vi "Redraw full indicator.vi"(8 "error in (no error)":errorcluster, 11 "D_Datagrid in":refnum<class "D_Datagrid.lvclass">) -> (0 "error out":errorcluster, 3 "D_Datagrid out":refnum<class "D_Datagrid.lvclass">)   [LabVIEW 2020, in "D Datagrid Library.lvlib" / "D_Datagrid.lvclass"]
doc: "Redraws the control to show the current DataElements value. If \"Auto Update Indicator\" is True, this is called automatically when writing DataElements. Otherwise, you should call this manually when you want to update the indicator."
uses:
  D_Datagrid.lvclass
  C:/Program Files/National Instruments/LabVIEW 2020/vi.lib/QSI/QControls/QControl Classes/Control/Control.lvclass
  C:/Program Files/National Instruments/LabVIEW 2020/vi.lib/QSI/QControls/QControl Classes/Table/Table.lvclass
  D_Datagrid.lvclass/D_Datagrid.ctl
  DatagridElement/DatagridElement.lvclass/DatagridElement.ctl
  <vilib>/Utility/miscctls.llb/LVRowAndColumnTypeDef.ctl
  DatagridElement/Read Cell font.vi
  DatagridElement/Read Enabled state.vi
  Read DataElements.vi
  DatagridElement/DatagridElement.lvclass
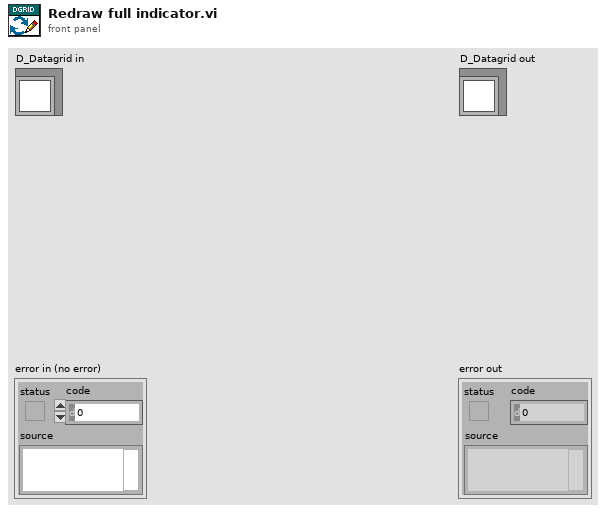
[diagram p1: front panel]
types:
  T1 = typedef "LVFontTypeDef.ctl" = cluster{"Font Name":string, "Size":u16, "Bold":bool, "Italic":bool, "Underline":bool, "Strikeout":bool, "Color":u32}
  T2 = enum8{"Enabled", "Disabled", "Disabled and Grayed Out"}
  T3 = cluster{"Accessors:Enabled state":enum8{"Enabled", "Disabled", "Disabled and Grayed Out"}, i32, i32}
  T4 = typedef "LVRowAndColumnTypeDef.ctl" = cluster{"Row":i32, "Column":i32}
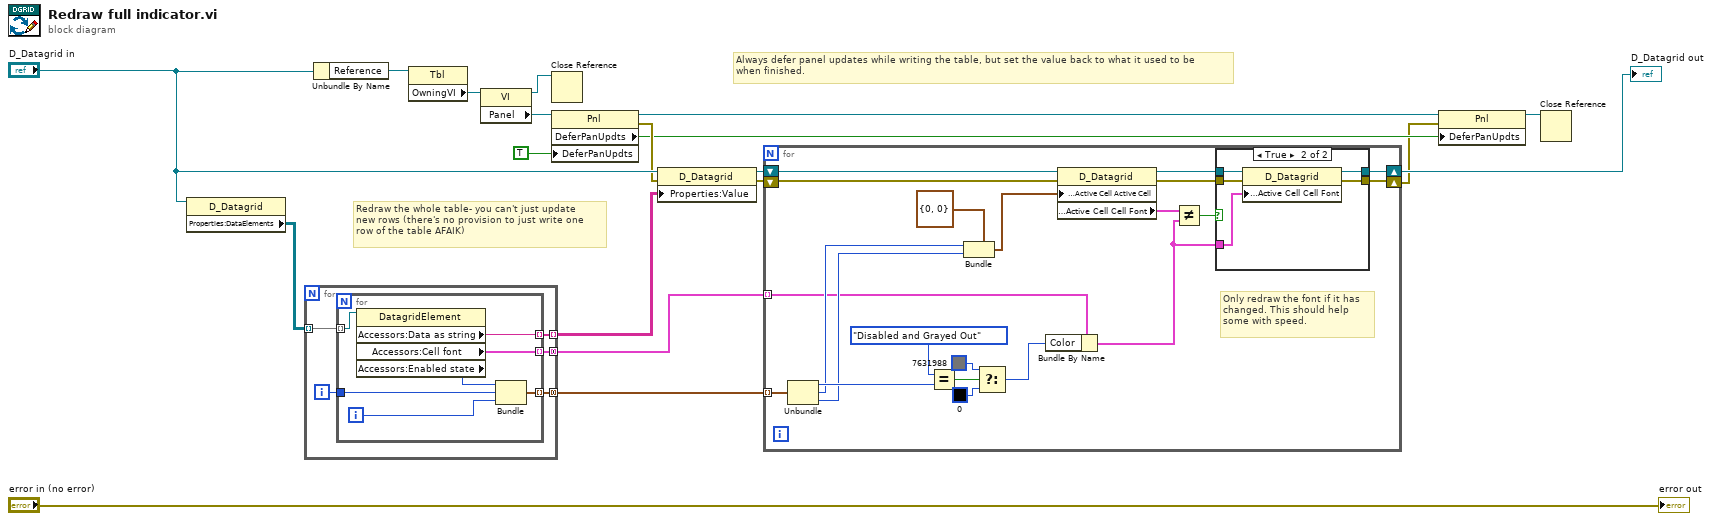
[diagram p0: block diagram]
diagram:
  # "Redraw the whole table- you can't just update\nnew rows (there's no provision to just write one\nrow of the table AFAIK)"
  # "Always defer panel updates while writing the table, but set the value back to what it used to be\nwhen finished."
  n1 = property class="D_Datagrid"(reference="D_Datagrid in") -> ("Properties:DataElements"=w4:refnum<class "DatagridElement.lvclass">[][])  [unwired: 1 in, 2 out]
  n2 = for {
    tunnel: w4 -> [w24] mode=indexing
    tunnel: [w23] -> w16 mode=indexing
    tunnel: [w21] -> w14 mode=concatenating
    tunnel: [w20] -> w1 mode=concatenating
    i -> [w22]
    n3 = for {
      tunnel: w24 -> [w31] mode=indexing
      tunnel: [w30] -> w23 mode=indexing
      tunnel: w22 -> [w29]
      tunnel: [w27] -> w21 mode=indexing
      tunnel: [w25] -> w20 mode=indexing
      i -> [w28]
      n4 = property class="DatagridElement"(reference=w31) -> ("Accessors:Data as string"=w30:string, "Accessors:Cell font"=w25:T1, "Accessors:Enabled state"=w26:T2)  [unwired: 1 in, 2 out]
      n5 = Bundle("Accessors:Enabled state"=w26, w29, w28) -> (w27:T3)  [unwired: 1 in]
    }
  }
  n6 = Unbundle By Name("D_Datagrid in") -> ("Reference"=w13:refnum<vi>)
  n7 = property class="Tbl"(reference=w13) -> ("OwningVI"=w12:refnum<vi>)  [unwired: 1 in, 2 out]
  n8 = property class="VI"(reference=w12) -> (reference out=w10:refnum<vi>, "Panel"=w6:refnum<vi>)  [unwired: 1 in, 1 out]
  n9 = Close Reference(reference=w10) -> ()  [unwired: 1 in, 1 out]
  n10 = property class="Pnl"(reference=w6, "DeferPanUpdts"=TRUE ("Defer Panel Updates")) -> (reference out=w9:refnum<vi>, error out=w11:errorcluster, "DeferPanUpdts"=w5:bool)  [unwired: 1 in]
  n11 = property class="D_Datagrid"(reference="D_Datagrid in", error in=w11, "Properties:Value"=w16) -> (reference out=w15:refnum<class "D_Datagrid.lvclass">, error out=w3:errorcluster)
  n12 = for {
    shift-right: [w40] -> w17
    shift-left: w15 -> [w52]
    tunnel: w14 -> [w51] mode=indexing
    shift-right: [w35] -> w2
    shift-left: w3 -> [w37]
    tunnel: w1 -> [w34] mode=indexing
    # "Only redraw the font if it has\nchanged. This should help\nsome with speed."
    n13 = Unbundle(w51) -> ("Accessors:Enabled state"=w50:T2, w44:i32, w43:i32)
    n14 = Equal?(x=T2."Disabled and Grayed Out" ("Accessors:Enabled state"), y=w50) -> (x = y?=w48:bool)
    n15 = Bundle(cluster=T4 {"Row"=0, "Column"=0} ("Active Cell:Active Cell"), "Row"=w44, "Column"=w43) -> (w45:T4)
    n16 = Select(t=u32 7631988, s=w48, f=u32 0) -> (s? t:f=w33:u32)
    n17 = Bundle By Name(cluster=w34, "Color"=w33) -> (w32:T1)
    n18 = property class="D_Datagrid"(reference=w52, error in=w37, "Properties:Active Cell Active Cell"=w45) -> (reference out=w41:refnum<class "D_Datagrid.lvclass">, error out=w36:errorcluster, "Properties:Active Cell Cell Font"=w39:T1)
    n19 = Not Equal?(x=w39, y=w32) -> (x != y?=w38:bool)
    n20 = case shown="True" w38 {
      tunnel: w41 -> [w54 w59]
      tunnel: [w54 w58] -> w40
      tunnel: w36 -> [w53 w57]
      tunnel: [w53 w56] -> w35
      tunnel: w32 -> [_ w55]
      frame False {
      }
      frame True {
        n21 = property class="D_Datagrid"(reference=w59, error in=w57, "Properties:Active Cell Cell Font"=w55) -> (reference out=w58:refnum<class "D_Datagrid.lvclass">, error out=w56:errorcluster)
      }
    }
  }
  "D_Datagrid out" <- w17
  n22 = property class="Pnl"(reference=w9, error in=w2, "DeferPanUpdts"=w5) -> (reference out=w8:refnum<vi>)  [unwired: 1 out]
  n23 = Close Reference(reference=w8) -> ()  [unwired: 1 in, 1 out]
  "error out" <- "error in (no error)"
